vi "replace class.vi"(10 "VI Path":path, 11 "qualified class name":string="tag bus.lvlib:data table.lvclass") -> ()   [LabVIEW 2013, in "scripting tools.lvlib"]
uses:
  <vilib>/Utility/traverseref.llb/TRef TravTarget.ctl
  scripting tools.lvlib
  <vilib>/Utility/traverseref.llb/VI Scripting - Traverse.lvlib
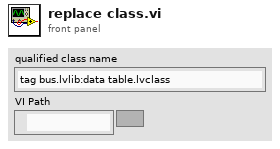
[diagram p1: front panel]
types:
  T1 = typedef "TRef TravTarget.ctl" = enum16{"FP", "BD", "Other"}
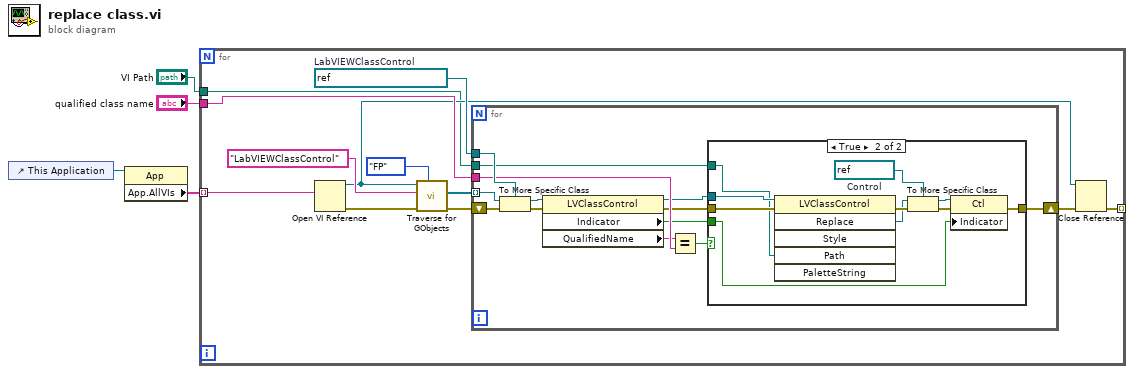
[diagram p0: block diagram]
diagram:
  n1 = control-ref of="This Application"() -> (w3:refnum<vi>)
  n2 = property class="App"(reference=w3) -> ("App.AllVIs"=w4:string[])  [unwired: 1 in, 2 out]
  n3 = for {
    tunnel: w4 -> [w16] mode=indexing
    tunnel: "qualified class name" -> [w9]
    tunnel: "VI Path" -> [w6]
    tunnel: [w5] -> _ mode=indexing
    w10 = refnum<vi> refnum  # LabVIEWClassControl
    n4 = Open VI Reference(vi path=w16) -> (vi reference=w8:refnum<vi>, error out=w15:errorcluster)  [unwired: 5 in]
    n5 = call <vilib>:"Traverse for GObjects.vi"("Traverse Target"=TRef_TravTarget."FP", "error in (no error)"=w15, "Class Name"="LabVIEWClassControl", "VI Refnum"=w8) -> ("error out"=w11:errorcluster, "References"=w12:refnum<vi>[])  [unwired: 4 in, 2 out]
    n6 = for {
      tunnel: w12 -> [w28] mode=indexing
      shift-right: [w18] -> w7
      shift-left: w11 -> [w29]
      tunnel: w10 -> [w27]
      tunnel: w9 -> [w24]
      tunnel: w6 -> [w17]
      n7 = To More Specific Class(target class=w27, reference=w28, error in=w29) -> (specific class reference=w26:refnum<vi>, error out=w25:errorcluster)
      n8 = property class="LVClassControl"(reference=w26, error in=w25) -> (reference out=w20:refnum<vi>, error out=w19:errorcluster, "Indicator"=w21:bool, "QualifiedName"=w23:string)
      n9 = Equal?(x=w23, y=w24) -> (x = y?=w22:bool)
      n10 = case shown="True" w22 {
        tunnel: w21 -> [_ w31]
        tunnel: w20 -> [_ w39]
        tunnel: w19 -> [w30 w40]
        tunnel: [w30 w36] -> w18
        tunnel: w17 -> [_ w38]
        frame False {
        }
        frame True {
          w32 = refnum<vi> refnum  # Control
          n11 = invoke class="LVClassControl" method="Replace"(reference=w39, error in=w40, "Path"=w38) -> (error out=w37:errorcluster, "Replace"=w34:refnum<vi>)  [unwired: 3 in, 4 out]
          n12 = To More Specific Class(target class=w32, reference=w34, error in=w37) -> (specific class reference=w33:refnum<vi>, error out=w35:errorcluster)
          n13 = property class="Ctl"(reference=w33, error in=w35, "Indicator"=w31) -> (error out=w36:errorcluster)  [unwired: 1 out]
        }
      }
    }
    n14 = Close Reference(reference=w8, error in (no error)=w7) -> (error out=w5:errorcluster)
  }
